vi "Get Next Trace ID.vi"(8 "error in (no error)":errorcluster, 11 "Trace Controller in":refnum<class "Trace Controller.lvclass">) -> (0 "error out":errorcluster, 2 "Next Trace ID":u64, 3 "Trace Controller out":refnum<class "Trace Controller.lvclass">)   [LabVIEW 2014, in "Robot Actor Framework.lvlib" / "Trace.lvlib" / "Trace Controller.lvclass"]
uses:
  Trace Controller.lvclass
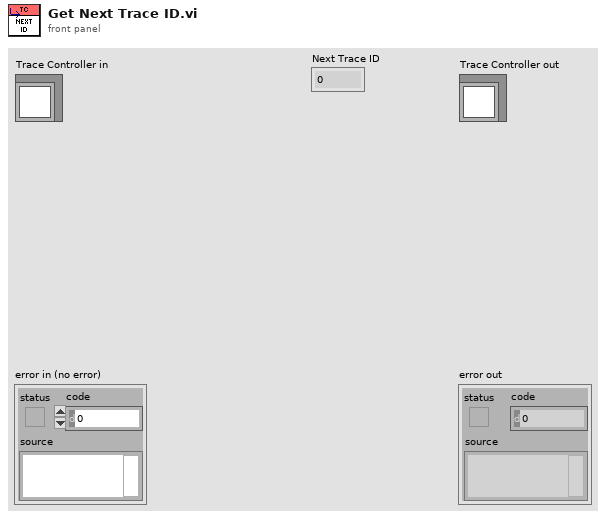
[diagram p1: front panel]
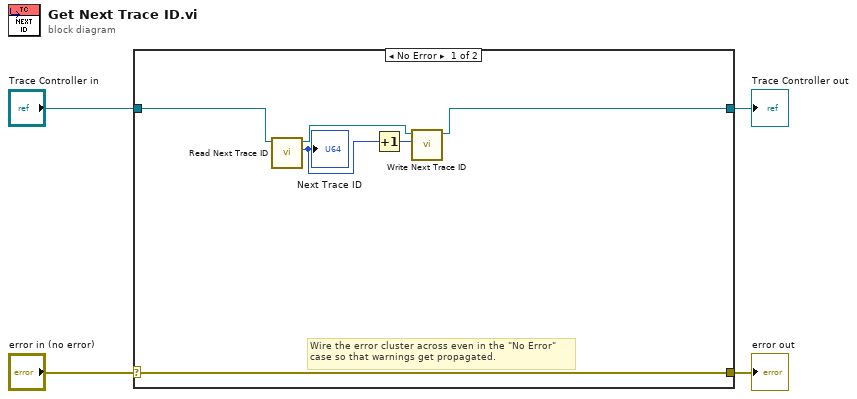
[diagram p0: block diagram]
diagram:
  n1 = case shown="No Error" "error in (no error)" {
    selector: "error in (no error)" -> [w10 w12]
    tunnel: [w10 w12] -> w3
    tunnel: [w7 w11] -> w1
    tunnel: "Trace Controller in" -> [w8 w11]
    frame No Error {
      # "Wire the error cluster across even in the \"No Error\"\ncase so that warnings get propagated."
      n2 = call-dynamic "Read Next Trace ID.vi"("Trace Controller in"=w8) -> ("Next Trace ID"=w6:u64, "Trace Controller out"=w9:refnum<class "Trace Controller.lvclass">)  [unwired: 8 in, 1 out]
      "Next Trace ID" <- w6
      n3 = Increment(x=w6) -> (x+1=w5:u64)
      n4 = call-dynamic "Write Next Trace ID.vi"("Next Trace ID"=w5, "Trace Controller in"=w9) -> ("Trace Controller out"=w7:refnum<class "Trace Controller.lvclass">)  [unwired: 8 in, 1 out]
    }
    frame Error {
    }
  }
  "error out" <- w3
  "Trace Controller out" <- w1
